vi "Get test names and limits.vi"(0 "Refnum in":T2, 5 "Variant":string, 9 "System data in":T1, 11 "error in":errorcluster) -> (4 "Refnum out":T2, 10 "System data out":T1, 15 "error out":errorcluster)   [LabVIEW 2023]
uses:
  <vilib>/Utility/config.llb/NI_LVConfig.lvlib
  <vilib>/Utility/config.llb/Read Key (String).vi
  <vilib>/Utility/config.llb/Config Data RefNum.ctl
  <vilib>/NI/Modbus Library/API/Master/Modbus Master.lvclass
  System Data.ctl
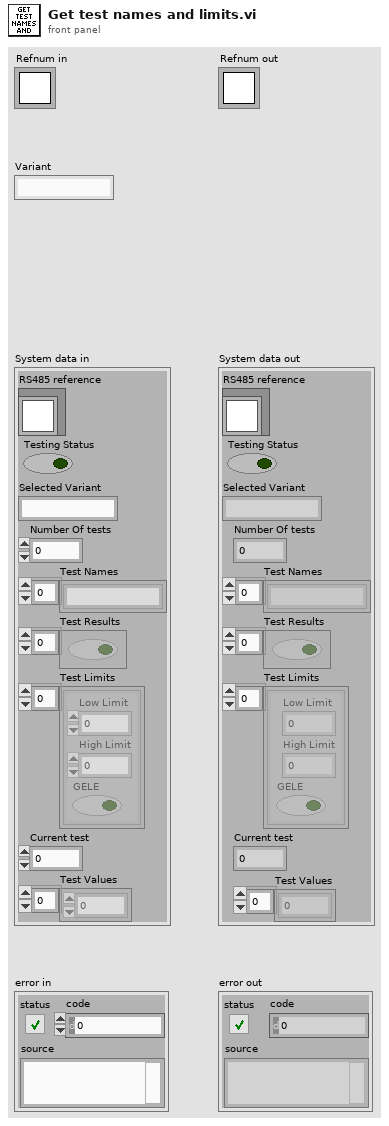
[diagram p1: front panel]
types:
  T1 = typedef "System Data.ctl" = cluster{"RS485 reference":refnum<class "Modbus Master.lvclass">, "Testing Status":bool, "Selected Variant":string, "Number Of tests":i32, "Test Names":string[], "Test Results":bool[], "Test Limits":cluster{"Low Limit":dbl, "High Limit":dbl, "GELE":bool}[], "Current test":i32, "Test Values":dbl[]}
  T2 = typedef "NI_LVConfig.lvlib/Config Data RefNum.ctl" = refnum<k1>
  T3 = cluster{"Low Limit":dbl, "High Limit":dbl, "GELE":bool}
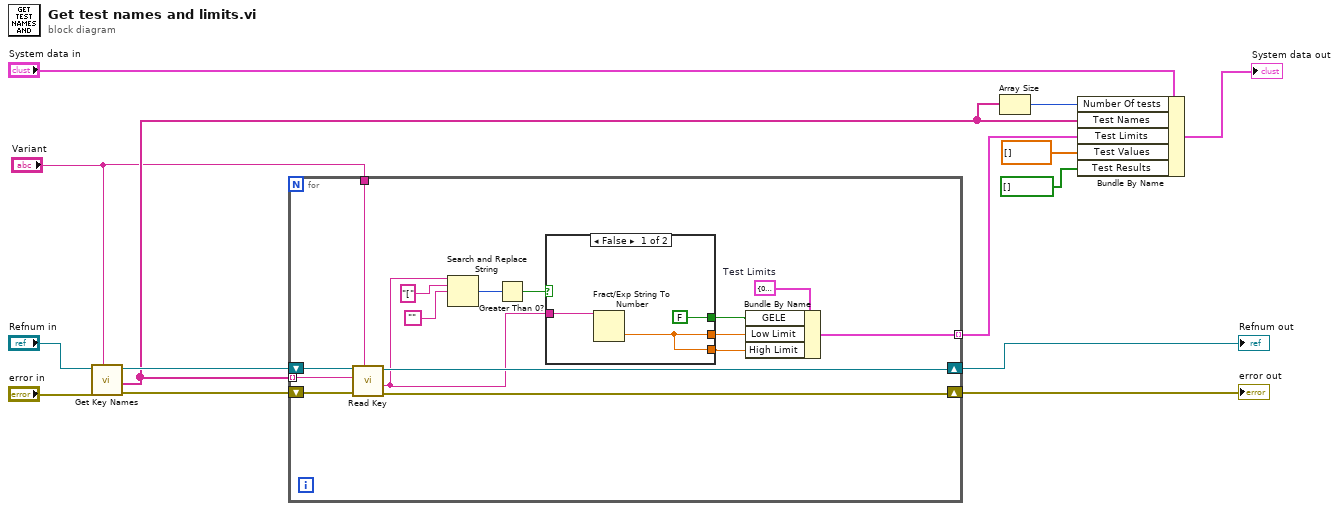
[diagram p0: block diagram]
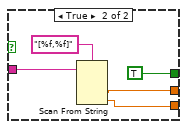
[diagram p2: hidden frame]
diagram:
  n1 = call <vilib>:"Get Key Names.vi"("section"="Variant", "error in (no error)"="error in", "refnum"="Refnum in") -> ("error out"=w11:errorcluster, "key names"=w6:string[], "refnum out"=w12:T2)  [unwired: 5 in, 1 out]
  n2 = for {
    shift-right: [w29] -> w9
    shift-left: w12 -> [w30]
    shift-right: [w26] -> w8
    shift-left: w11 -> [w27]
    tunnel: "Variant" -> [w28]
    tunnel: w6 -> [w25] mode=indexing
    tunnel: [w18] -> w10 mode=indexing
    w19 = T3 {"Low Limit"=0.0, "High Limit"=0.0, "GELE"=FALSE}  # Test Limits
    n3 = call-poly <vilib>:"Read Key.vi"("section"=w28, "error in (no error)"=w27, "key"=w25, "refnum"=w30) -> ("error out"=w26:errorcluster, "value"=w24:string, "refnum out"=w29:T2)  [unwired: 4 in, 1 out]
    n4 = Search and Replace String(input string=w24, search string="[", replace string="") -> (number of replacements=w21:i32)  [unwired: 5 in, 3 out]
    n5 = Greater Than 0?(x=w21) -> (x > 0?=w20:bool)
    n6 = case shown="False" w20 {
      tunnel: w24 -> [w33 w37]
      tunnel: [w31 w36] -> w17
      tunnel: [w31 w35] -> w16
      tunnel: [FALSE ("GELE") TRUE ("GELE")] -> w15
      frame False {
        n7 = Fract/Exp String To Number(string=w33) -> (number=w31:dbl)  [unwired: 3 in, 1 out]
      }
      frame True {
        n8 = Scan From String(format string="[%f,%f]", input string=w37) -> (output 1=w36:dbl, output 2=w35:dbl)  [unwired: 4 in, 3 out]
      }
    }
    n9 = Bundle By Name(cluster=w19, "GELE"=w15, "Low Limit"=w17, "High Limit"=w16) -> (w18:T3)
  }
  "error out" <- w8
  "Refnum out" <- w9
  n10 = Array Size(array=w6) -> (size(s)=w5:i32)
  n11 = Bundle By Name(cluster="System data in", "Number Of tests"=w5, "Test Names"=w6, "Test Limits"=w10, "Test Values"=dbl[] [], "Test Results"=bool[] []) -> (→"System data out":T1)
